vi "ModifyAttribute.vi"(0 "reference in":refnum<class "G#BaseClass1.lvclass">, 1 "Lock time (ms)":u32, 5 "error in (no error)":errorcluster) -> (14 "reference out":refnum<class "G#BaseClass1.lvclass">, 19 "error out":errorcluster)   [LabVIEW 2010, in "G#BaseClass1.lvclass"]
uses:
  G#BaseClass1.lvclass
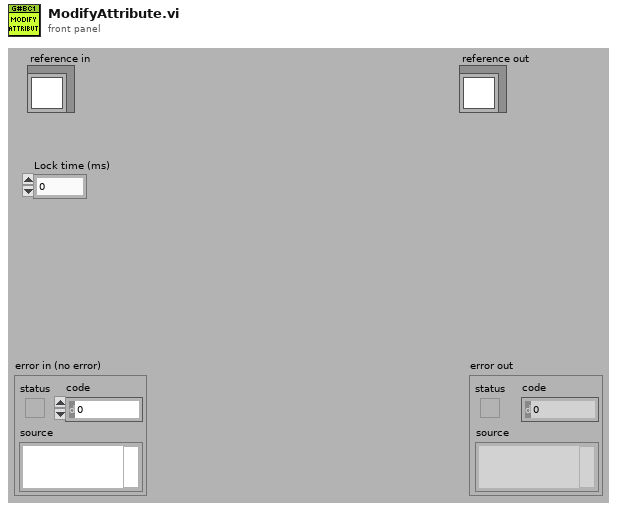
[diagram p1: front panel]
types:
  T1 = typedef "G#BaseClass1.lvclass/ObjectAttributesRef.ctl" = refnum<data-value>
  T2 = typedef "G#BaseClass1.lvclass/ObjectAttributes.ctl" = cluster{"Numeric":dbl, "Array":dbl[]}
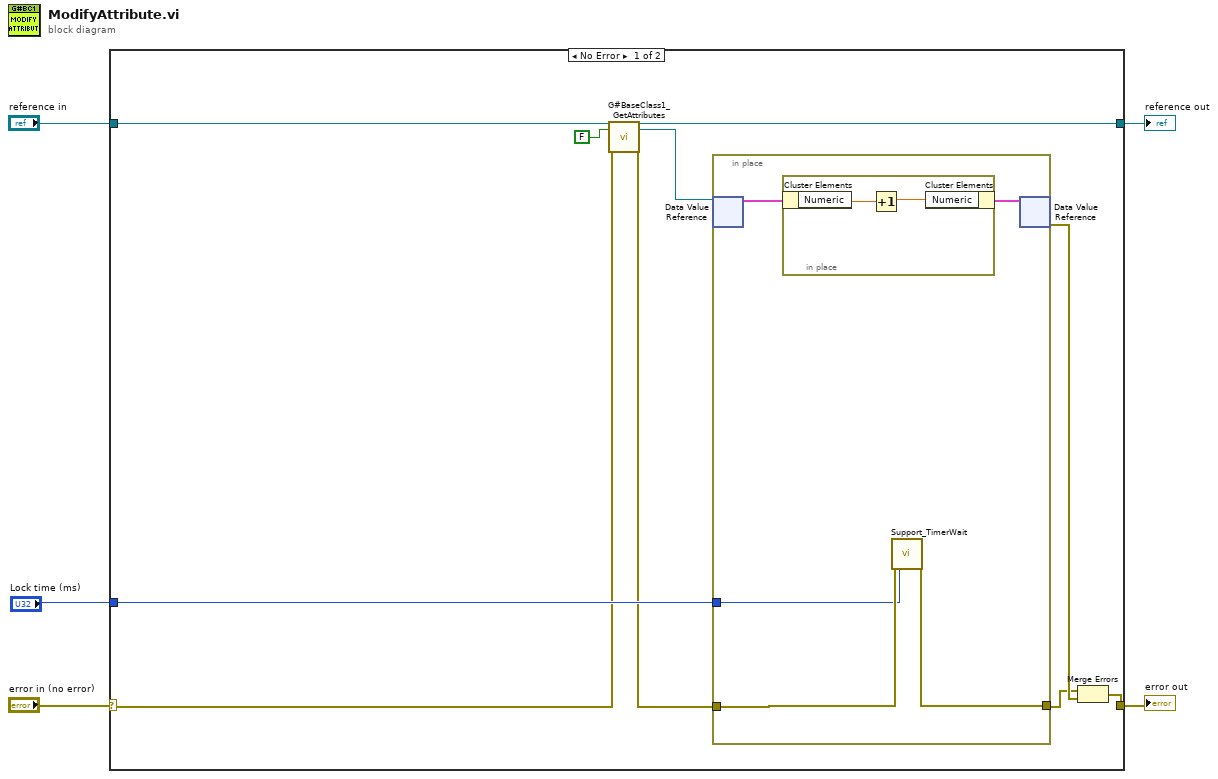
[diagram p0: block diagram]
diagram:
  n1 = case shown="No Error" "error in (no error)" {
    selector: "error in (no error)" -> [w7 w24]
    tunnel: [w15 w24] -> w4
    tunnel: [w10 w23] -> w2
    tunnel: "reference in" -> [w11 w23]
    tunnel: "Lock time (ms)" -> [w12 _]
    frame No Error {
      n2 = call "G#BaseClass1_GetAttributes.vi"("reference in"=w11, "return data? (T)"=FALSE, "error in (no error)"=w7) -> ("reference out"=w10:refnum<class "G#BaseClass1.lvclass">, "attributes ref"=w9:T1, "error out"=w6:errorcluster)  [unwired: 13 in, 1 out]
      n3 = in-place {
        in-place-border: w6 -> [w18]
        in-place-border: [w17] -> w13
        in-place-border: w12 -> [w16]
        n4 = in-place-dvr #1(w9) -> (w19:T2)  [unwired: 1 out]
        n5 = in-place {
          n6 = in-place-cluster #2(w19) -> ("Numeric"=w22:dbl)
          n7 = Increment(x=w22) -> (x+1=w21:dbl)
          n8 = in-place-cluster #2("Numeric"=w21) -> (w20:T2)
        }
        n9 = call "Support_TimerWait.vi"("error in (no error)"=w18, "milliseconds to wait"=w16) -> ("error out"=w17:errorcluster)  [unwired: 17 in]
        n10 = in-place-dvr #1(w20) -> (w14:errorcluster)  [unwired: 1 out]
      }
      n11 = Merge Errors(w13, w14) -> (w15:errorcluster)
    }
    frame Error {
    }
  }
  "error out" <- w4
  "reference out" <- w2
